vi "Demo.vi"() -> ()   [LabVIEW 2018, in "Queue.lvlib"]
uses:
  Queue.lvlib
  ff152fcc-b31c-470d-af7e-81e9149920c3.vi
  3a8111e8-9793-4339-bc31-099fb7087c15.vi
  cbda833d-b843-47c6-901d-fad0553c39ee.vi
  21de42a5-3b39-4ac6-9af5-8886f64cdfe3.vi
  411f2538-55e3-4a37-bdc6-b30b308c6804.vi
  d23851c3-c178-4ea2-93a5-d675b1bcab8b.vi
  4becfa95-8fea-4955-886a-6edb3b8740ea.vi
  3e7329be-45d5-4a20-94c7-c4a4647cfab4.vi
  111c9c86-2e6b-4769-81f6-ef509a265678.vi
  955eceb6-4673-4f8e-b0ba-f9eafbb93845.vi
  610312e2-ffa9-433b-b24d-b96227872030.vi
panel:
  out "Error":errorcluster
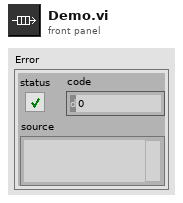
[diagram p1: front panel]
types:
  T1 = enum16{"invalid", "init", "pause", "more", "more2"}[]
  T2 = cluster{"Queue out":refnum<queue>, "Queue out":refnum<queue>}
  T3 = enum16{"invalid", "init", "pause", "exit", "more2"}
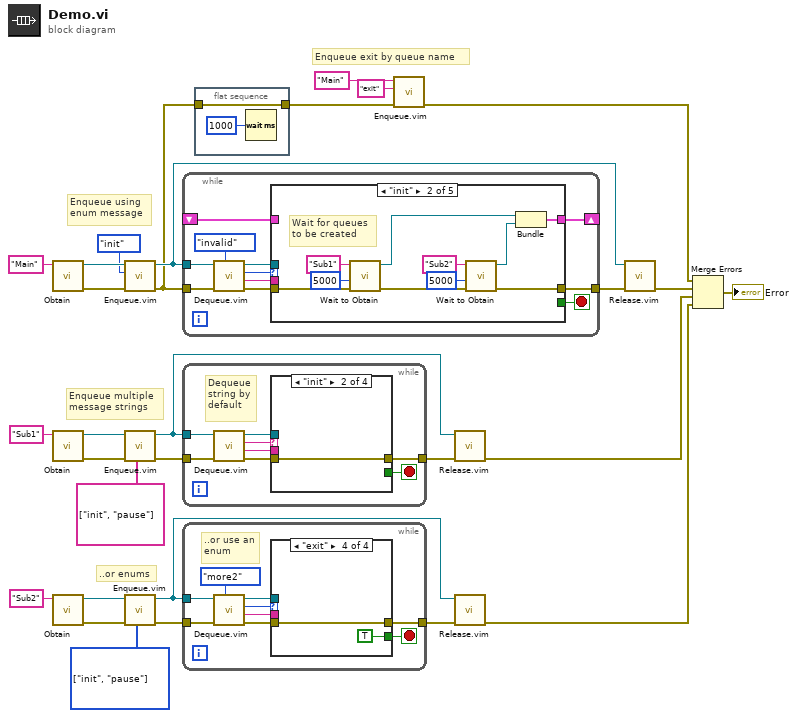
[diagram p0: block diagram]
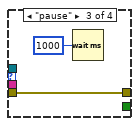
[diagram p4: hidden frame]
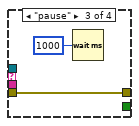
[diagram p6: hidden frame]
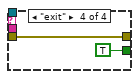
[diagram p7: hidden frame]
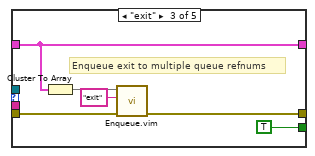
[diagram p9: hidden frame]
diagram:
  w13 = T1 [enum."init", enum."pause"] items=["invalid", "init", "pause", "more", "more2"] ("Messages")
  # "..or enums"
  # "Enqueue multiple\nmessage strings"
  # "Enqueue using\nenum message"
  # "Enqueue exit by queue name"
  n1 = call "Obtain.vi"("Queue Name (\"\"=Unnamed)"="Main" ("Queue Name (\"\"=Unnamed)")) -> ("error out"=w20:errorcluster, "Queue out"=w19:refnum<queue>)  [unwired: 8 in, 1 out]
  n2 = call "Obtain.vi"("Queue Name (\"\"=Unnamed)"="Sub1" ("Queue Name (\"\"=Unnamed)")) -> ("error out"=w27:errorcluster, "Queue out"=w28:refnum<queue>)  [unwired: 8 in, 1 out]
  n3 = call "Obtain.vi"("Queue Name (\"\"=Unnamed)"="Sub2" ("Queue Name (\"\"=Unnamed)")) -> ("error out"=w12:errorcluster, "Queue out"=w11:refnum<queue>)  [unwired: 8 in, 1 out]
  n4 = call "Enqueue.vim"("error in (no error)"=w20, "Message"=enum16{"invalid", "init", "wait", "exit"}."init", "Queue in"=w19) -> ("error out"=w7:errorcluster, "Queue out"=w22:refnum<queue>)  [unwired: 7 in]
  n5 = call "Enqueue.vim"("Messages"=string[] ["init", "pause"], "error in (no error)"=w27, "Queue in"=w28) -> ("error out"=w25:errorcluster, "Queue out"=w23:refnum<queue>)  [unwired: 7 in]
  n6 = call "Enqueue.vim"("Messages"=w13, "error in (no error)"=w12, "Queue in"=w11) -> ("error out"=w14:errorcluster, "Queue out"=w16:refnum<queue>)  [unwired: 7 in]
  n7 = while {
    tunnel: w7 -> [w40]
    tunnel: w22 -> [w39]
    tunnel: [w36] -> w21
    shift-right: [w31] -> _
    shift-left: _ -> [w30]
    stop <- w33 stop-if-true
    n8 = call "Dequeue.vim"("Message Type"=enum16{"invalid", "init", "wait", "exit"}."invalid", "error in (no error)"=w40, "Queue in"=w39) -> ("error out"=w35:errorcluster, "Data"=w37:string, "Message"=w38:enum16{"invalid", "init", "wait", "exit"}, "Queue out"=w34:refnum<queue>)  [unwired: 3 in, 2 out]
    n9 = case shown="\"init\"" w38 {
      tunnel: w37 -> [_ _ _ _ _]
      tunnel: [w42 w48 w56 w60 w62] -> w36
      tunnel: w35 -> [w42 w52 w55 w60 w62]
      tunnel: w34 -> [_ _ _ _ _]
      tunnel: [_ _ TRUE _ _] -> w33
      tunnel: [w41 w45 w57 w59 w61] -> w31
      tunnel: w30 -> [w41 _ w57 w59 w61]
      frame Default {
      }
      frame "init" {
        # "Wait for queues\nto be created"
        n10 = call "Wait to Obtain.vi"("error in (no error)"=w52, "Timeout in ms (5000)"=u32 5000, "Queue Name"="Sub1") -> ("error out"=w49:errorcluster, "Queue out"=w47:refnum<queue>)  [unwired: 6 in, 1 out]
        n11 = call "Wait to Obtain.vi"("error in (no error)"=w49, "Timeout in ms (5000)"=u32 5000, "Queue Name"="Sub2") -> ("error out"=w48:errorcluster, "Queue out"=w46:refnum<queue>)  [unwired: 6 in, 1 out]
        n12 = Bundle("Queue out"=w47, "Queue out"=w46) -> (w45:T2)  [unwired: 1 in]
      }
      frame "exit" {
        # "Enqueue exit to multiple queue refnums"
        n13 = Cluster To Array(cluster=w57) -> (array=w54:refnum<queue>[])
        n14 = call "Enqueue.vim"("error in (no error)"=w55, "Message"="exit", "Queue in"=w54) -> ("error out"=w56:errorcluster)  [unwired: 7 in, 1 out]
      }
      frame "wait" {
      }
      frame "invalid" {
      }
    }
  }
  n15 = while {
    tunnel: w25 -> [w70]
    tunnel: w23 -> [w69]
    tunnel: [w66] -> w24
    stop <- w63 stop-if-true
    # "Dequeue\nstring by\ndefault"
    n16 = call "Dequeue.vim"("error in (no error)"=w70, "Queue in"=w69) -> ("error out"=w65:errorcluster, "Data"=w67:string, "Message"=w68:string, "Queue out"=w64:refnum<queue>)  [unwired: 4 in, 2 out]
    n17 = case shown="\"init\"" w68 {
      tunnel: w67 -> [_ _ _ _]
      tunnel: [w71 w72 w74 w76] -> w66
      tunnel: w65 -> [w71 w72 w74 w76]
      tunnel: w64 -> [_ _ _ _]
      tunnel: [_ _ _ TRUE] -> w63
      frame Default {
      }
      frame "init" {
      }
      frame "pause" {
        n18 = Wait (ms)(milliseconds to wait=u32 1000) -> ()  [unwired: 1 out]
      }
      frame "exit" {
      }
    }
  }
  n19 = while {
    tunnel: w14 -> [w85]
    tunnel: w16 -> [w84]
    tunnel: [w81] -> w15
    stop <- w78 stop-if-true
    # "..or use an\nenum"
    n20 = call "Dequeue.vim"("Message Type"=T3."more2", "error in (no error)"=w85, "Queue in"=w84) -> ("error out"=w80:errorcluster, "Data"=w82:string, "Message"=w83:T3, "Queue out"=w79:refnum<queue>)  [unwired: 3 in, 2 out]
    n21 = case shown="\"exit\"" w83 {
      tunnel: w82 -> [_ _ _ _]
      tunnel: [w86 w87 w89 w91] -> w81
      tunnel: w80 -> [w86 w87 w89 w91]
      tunnel: w79 -> [_ _ _ _]
      tunnel: [_ _ _ TRUE] -> w78
      frame Default {
      }
      frame "init" {
      }
      frame "pause" {
        n22 = Wait (ms)(milliseconds to wait=u32 1000) -> ()  [unwired: 1 out]
      }
      frame "exit" {
      }
    }
  }
  n23 = flat-sequence {
    tunnel: w7 -> [w92]
    tunnel: [w92] -> w6
    frame #0 {
      n24 = Wait (ms)(milliseconds to wait=u32 1000) -> ()  [unwired: 1 out]
    }
  }
  n25 = call "Enqueue.vim"("error in (no error)"=w6, "Message"="exit", "Queue in"="Main") -> ("error out"=w4:errorcluster)  [unwired: 7 in, 1 out]
  n26 = call "Release.vim"("error in (no error)"=w24, "Queue in"=w23) -> ("error out"=w3:errorcluster)  [unwired: 7 in, 2 out]
  n27 = call "Release.vim"("error in (no error)"=w15, "Queue in"=w16) -> ("error out"=w2:errorcluster)  [unwired: 7 in, 2 out]
  n28 = call "Release.vim"("error in (no error)"=w21, "Queue in"=w22) -> ("error out"=w5:errorcluster)  [unwired: 7 in, 2 out]
  n29 = Merge Errors(w4, w5, w3, w2) -> (→"Error":errorcluster)
